vi "Send.vi"(8 "error in":errorcluster, 11 "Segmented Upload Transfer":refnum<class "Segmented Upload Transfer.lvclass">) -> (0 "error out":errorcluster, 3 "Segmented Upload Transfer":refnum<class "Segmented Upload Transfer.lvclass">)   [LabVIEW 2020, in "SDO Manager.lvlib" / "Segmented Upload Transfer.lvclass"]
doc: "Service SDO upload\nThe client is using the service SDO upload for transferring the data from the server (owner of the\nobject dictionary) to the client."
uses:
  Segmented Upload Transfer.lvclass
  Segmented Upload Transfer.lvclass/Segmented Upload Transfer.ctl
  HAL/Source/Interfaces/ICommunicate/ICommunicate.lvclass
  CANopen Message/CANopen Message.lvclass
  D:/git/CANopen-LabVIEW/source/SDO Manager/SDO Transfer/SDO Transfer.lvclass
  D:/git/CANopen-LabVIEW/source/SDO Manager/Segmented Upload Transfer/Segmented Upload Transfer.lvclass
  Typedefs/Function Code.ctl
  CANopen.lvlib
  SDO Transfer/SDO Transfer.lvclass
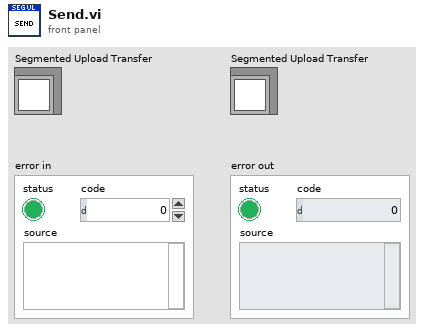
[diagram p1: front panel]
types:
  T1 = typedef "CANopen.lvlib/Function Code.ctl" = u8
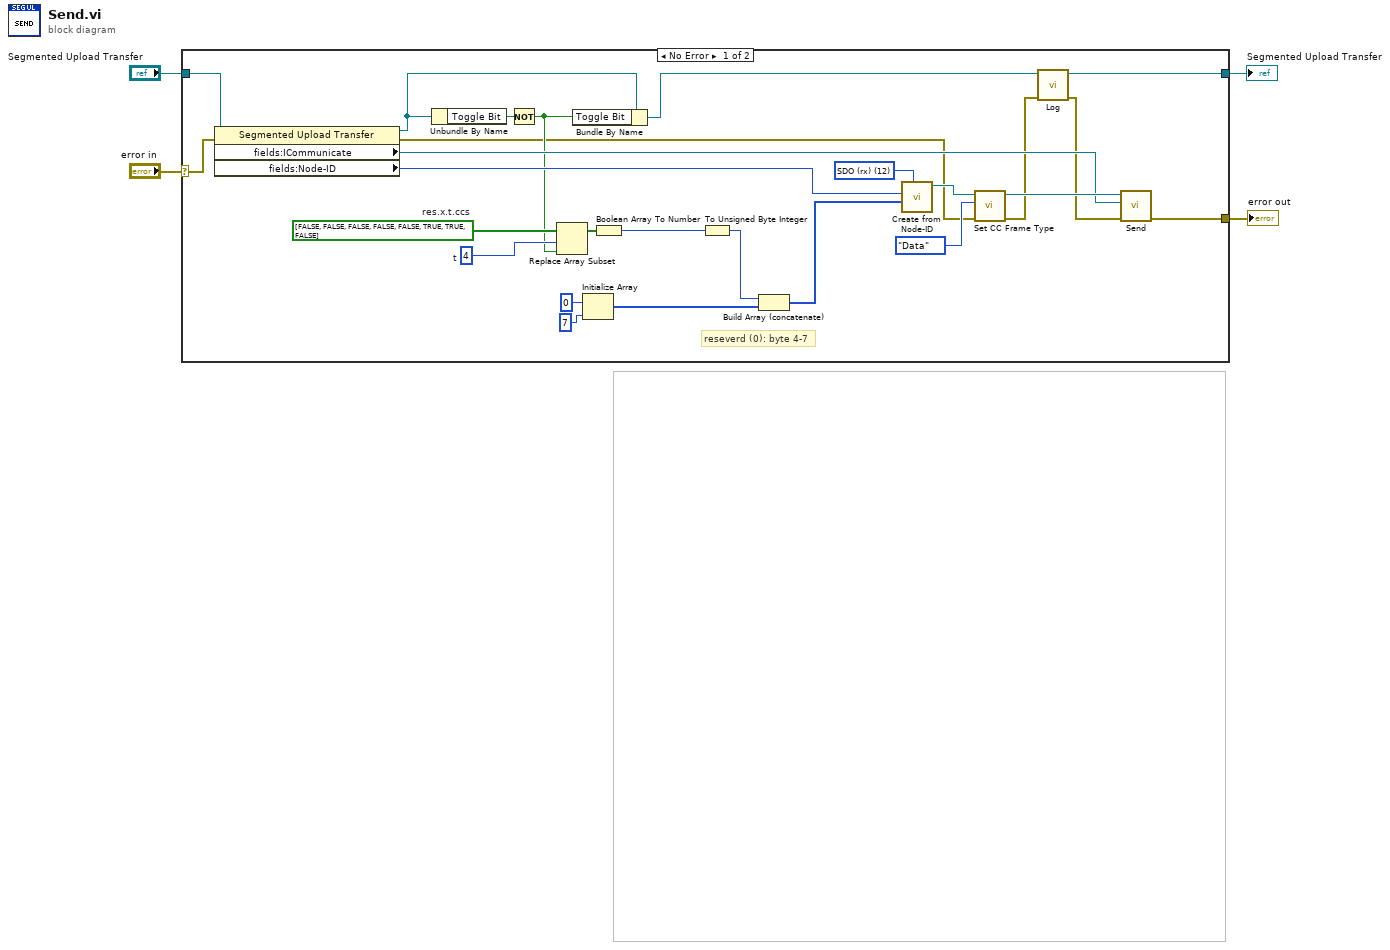
[diagram p0: block diagram]
diagram:
  n1 = case shown="No Error" "error in" {
    selector: "error in" -> [w30 w31]
    tunnel: "Segmented Upload Transfer" -> [w29 w32]
    tunnel: [w7 w32] -> w2
    tunnel: [w18 w31] -> w1
    frame No Error {
      w15 = 4  # t
      w16 = bool[] [FALSE, FALSE, FALSE, FALSE, FALSE, TRUE, TRUE, FALSE]  # res.x.t.ccs
      w24 = T1 12 items=["NMT"=0, "EMCY/SYNC"=1, "TIME"=2, "PDO1 (tx)"=3, "PDO1 (rx)"=4, "PDO2 (tx)"=5, "PDO2 (rx)"=6, "PDO3 (tx)"=7, "PDO3 (rx)"=8, "PDO4 (tx)"=9, "PDO4 (rx)"=10, "SDO (tx)"=11, "SDO (rx)"=12, "NMT error control"=14] ("Function Code")
      # "reseverd (0): byte 4-7"
      n2 = property class="Segmented Upload Transfer"(reference=w29, error in=w30) -> (reference out=w17:refnum<class "Segmented Upload Transfer.lvclass">, error out=w8:errorcluster, "fields:ICommunicate"=w19:refnum<class "ICommunicate.lvclass">, "fields:Node-ID"=w28:u8)
      n3 = Unbundle By Name(w17) -> ("Toggle Bit"=w14:bool)
      n4 = Not(x=w14) -> (.not. x?=w10:bool)
      n5 = Replace Array Subset(array=w16, new element=w10, index=w15) -> (w13:bool[])
      n6 = Bundle By Name(cluster=w17, "Toggle Bit"=w10) -> (w9:refnum<class "Segmented Upload Transfer.lvclass">)
      n7 = Initialize Array(u8 0, 7 ("y")) -> (w27:u8[])
      n8 = Boolean Array To Number(Boolean array=w13) -> (number=w12:u32)
      n9 = To Unsigned Byte Integer(number=w12) -> (unsigned 8bit integer=w11:u8)
      n10 = Build Array (concatenate)(w11, w27) -> (w25:u8[])
      n11 = call "Create from Node-ID.vi"("Function Code"=w24, "Data"=w25, "Node-ID"=w28) -> ("CANopen Message"=w23:refnum<class "CANopen Message.lvclass">)  [unwired: 8 in]
      n12 = call "Set CC Frame Type.vi"("error in"=w8, "CC Frame Type"=enum8{"Data", "Remote", "Error", "Overload"}."Data", "CANopen Message in"=w23) -> ("error out"=w6:errorcluster, "CANopen Message out"=w22:refnum<class "CANopen Message.lvclass">)  [unwired: 7 in]
      n13 = call "Log.vi"("error in"=w6, "SDO Transfer in"=w9) -> ("error out"=w5:errorcluster, "SDO Transfer out"=w7:refnum<class "Segmented Upload Transfer.lvclass">)  [unwired: 8 in]
      n14 = call "Send.vi"("error in"=w5, "ICommunicate"=w19, "CANopen Message in"=w22) -> ("error out"=w18:errorcluster)  [unwired: 7 in, 1 out]
    }
    frame Error {
    }
  }
  "Segmented Upload Transfer" <- w2
  "error out" <- w1
